vi "Renishaw-XL80_SetMatCompFactor.vi"(8 "error in (no error)":errorcluster, 10 "MatCompFactor":dbl, 11 "Renishaw-XL80_EMU in":refnum<class "Renishaw-XL80_EMU.lvclass">) -> (0 "error out":errorcluster, 3 "Renishaw-XL80_EMU out":refnum<class "Renishaw-XL80_EMU.lvclass">)   [LabVIEW 2024, in "Renishaw-XL80_EMU.lvclass"]
doc: "Writing this property will set the material compensation factor.\n\nDefinition\nput_MatCompFactor ( [in] double newVal);\nParameters\nnewVal\nSpecifies the material compensation factor to use.\n\nComments\nThis property will return with an HRESULT of E_FAIL if the client has set AutoCompensationMode to AUTO_COMPENSATION_FULL. This warns the client that setting the material compensation factor whilst it is being automatically updated is somewhat pointless. Otherwise it will return an HRESULT of S_OK.\n\nThe material compensation factor is a factor which when multiplied by the raw laser measurement will compensate the reading for thermal growth of the material, thereby estimating the reading that would be obtained if the material temperature had been 20°C. Note that MatCompFactor is a value very close to 1.00. For example if the expansion coefficient is set to 10ppm/°C and the current material temperature is 25°C then MatCompFactor will be 0.9999"
uses:
  Renishaw-XL80_EMU.lvclass
  Renishaw-XL80_EMU.lvclass/Renishaw-XL80_EMU.ctl
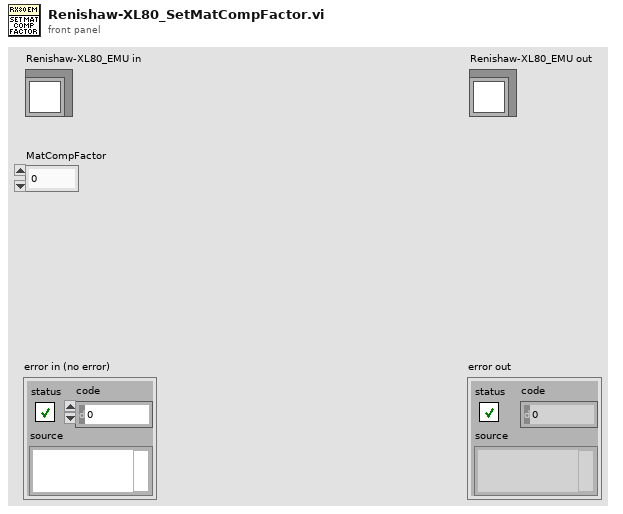
[diagram p1: front panel]
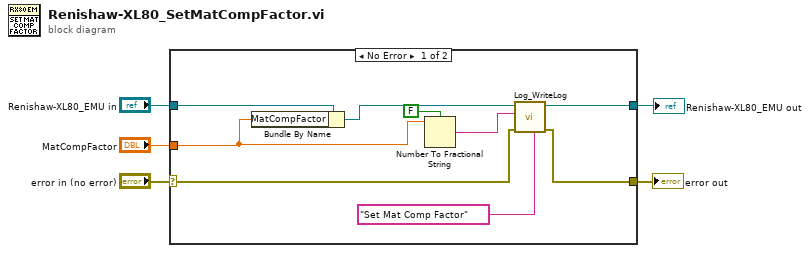
[diagram p0: block diagram]
diagram:
  n1 = case shown="No Error" "error in (no error)" {
    selector: "error in (no error)" -> [w8 w16]
    tunnel: [w7 w16] -> w4
    tunnel: "Renishaw-XL80_EMU in" -> [w14 w15]
    tunnel: [w9 w15] -> w2
    tunnel: "MatCompFactor" -> [w6 _]
    frame No Error {
      n2 = Bundle By Name(cluster=w14, "MatCompFactor"=w6) -> (w10:refnum<class "Renishaw-XL80_EMU.lvclass">)
      n3 = Number To Fractional String(use system decimal point (T)=FALSE, number=w6) -> (F-format string=w13:string)  [unwired: 2 in]
      n4 = call-dynamic "Log_WriteLog.vi"("Additional text"="Set Mat Comp Factor", "error in (no error)"=w8, "Command"=w13, "Log in"=w10) -> ("error out"=w7:errorcluster, "Log out"=w9:refnum<class "Renishaw-XL80_EMU.lvclass">)  [unwired: 6 in]
    }
    frame Error {
    }
  }
  "error out" <- w4
  "Renishaw-XL80_EMU out" <- w2
